vi "TEST ONLY - Core Wrapper.vi"(8 "error in (no error)":errorcluster, 11 "Ex Nested in":refnum<class "SuperClass.lvclass">) -> (0 "error out":errorcluster)   [LabVIEW 2014, in "SuperClass.lvclass"]
uses:
  SuperClass.lvclass
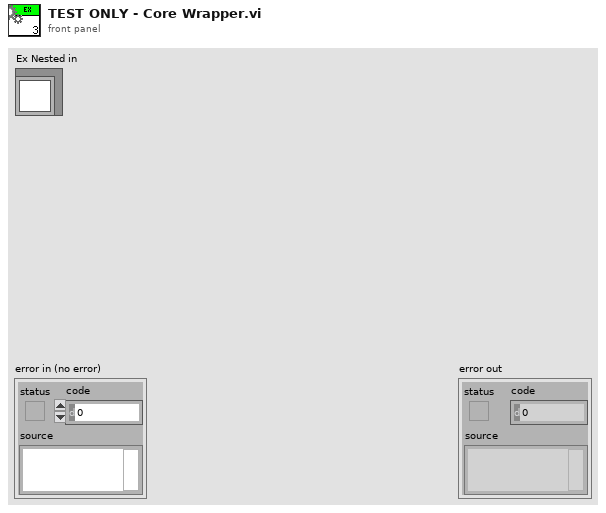
[diagram p1: front panel]
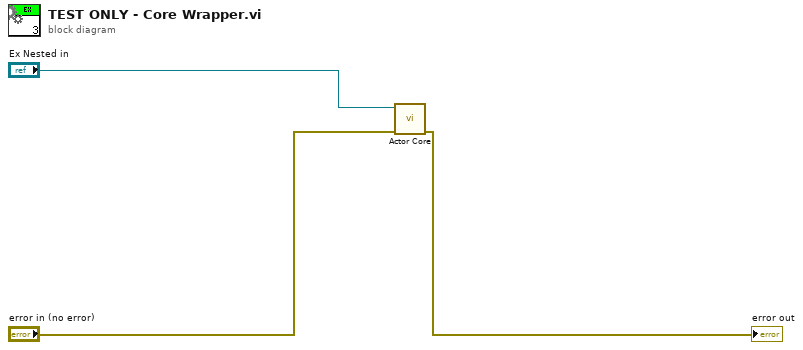
[diagram p0: block diagram]
diagram:
  n1 = call-dynamic "Actor Core.vi"("error in"="error in (no error)", "Actor in"="Ex Nested in") -> ("error out"=→"error out":errorcluster)  [unwired: 8 in, 1 out]
